vi "Initialize.vi"(8 "error in (no error)":errorcluster, 9 "Ethernet Config":T1={"IP Address"=[192, 168, 0, 1], "Port No"=24691}, 11 "Device ID (0)":i32) -> (0 "error out":errorcluster, 3 "Device ID out":i32)   [LabVIEW 2014, in "KEYENCE LJ-X8000A.lvlib"]
doc: "Establishes communication with the instrument and optionally performs an instrument identification query and/or an instrument reset. It also places the instrument in a default state needed for other instrument driver operations. Therefore, call this VI before calling other instrument driver VIs for this instrument. Generally, you need to call the <b>Initialize</b> VI only once at the beginning of an application."
uses:
  KEYENCE LJ-X8000A.lvlib
  Clusters/Ethernet Config.ctl
panel:
  # "(c) 2019 KEYENCE CORPORATION.  ALL RIGHTS RESERVED."
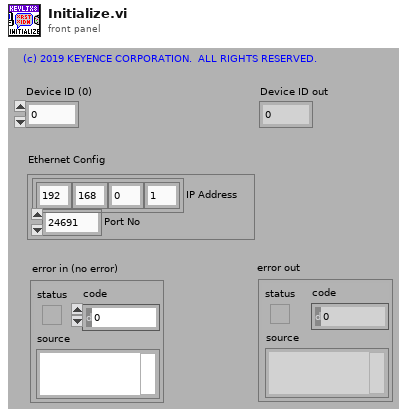
[diagram p1: front panel]
types:
  T1 = typedef "KEYENCE LJ-X8000A.lvlib/Ethernet Config.ctl" = cluster{"IP Address":u8[], "Port No":u16}
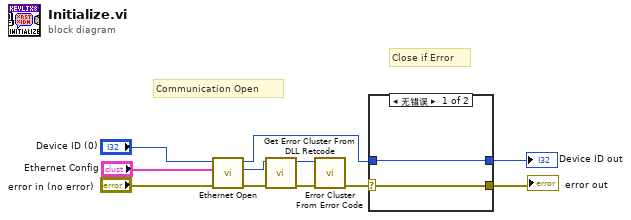
[diagram p0: block diagram]
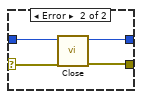
[diagram p2: hidden frame]
diagram:
  # "Close if Error"
  # "Communication Open"
  n1 = call "Ethernet Open.vi"("error in (no error)"="error in (no error)", "Ethernet Config"="Ethernet Config", "Device ID (0)"="Device ID (0)") -> ("error out"=w8:errorcluster, "Return Code"=w7:i32, "Device ID out"=w5:i32)  [unwired: 6 in]
  n2 = call "Get Error Cluster From DLL Retcode.vi"("error in (no error)"=w8, "DLL Return Code"=w7) -> ("error out"=w4:errorcluster, "VI Error Code"=w1:i32)  [unwired: 8 in]
  n3 = call <vilib>:"Error Cluster From Error Code.vi"("error in (no error)"=w4, "error code (0)"=w1) -> ("error out"=w2:errorcluster)  [unwired: 7 in]
  n4 = case shown="无错误" w2 {
    selector: w2 -> [w13 w17]
    tunnel: [w13 w16] -> w6
    tunnel: w5 -> [w12 w15]
    tunnel: [w12 w14] -> w3
    frame No Error {
    }
    frame Error {
      n5 = call "Close.vi"("error in (no error)"=w17, "Device ID (0)"=w15) -> ("error out"=w16:errorcluster, "Device ID out"=w14:i32)  [unwired: 8 in]
    }
  }
  "error out" <- w6
  "Device ID out" <- w3
